vi "set_ready.vi"(8 "error in (no error)":errorcluster, 10 "ready?":bool, 11 "ErrorController in":refnum<class "ErrorController.lvclass">) -> (0 "error out":errorcluster, 3 "ErrorController out":refnum<class "ErrorController.lvclass">)   [LabVIEW 2010, in "ErrorController.lvclass"]
uses:
  ErrorController.lvclass
  ErrorController.lvclass/ErrorController.ctl
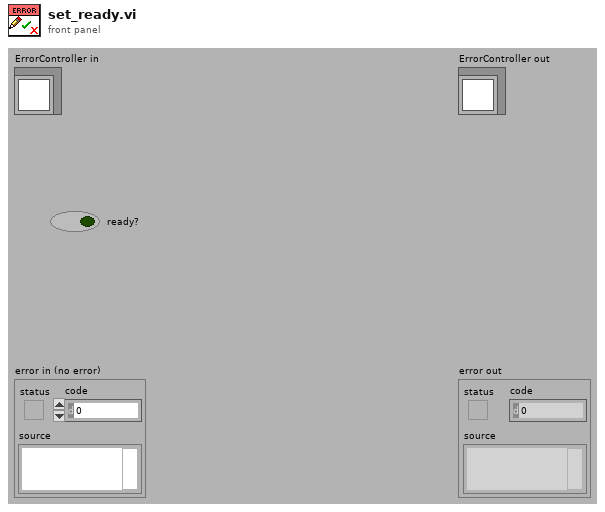
[diagram p1: front panel]
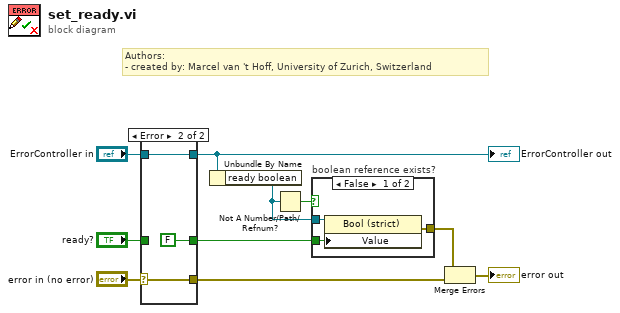
[diagram p0: block diagram]
diagram:
  # "Authors: \n- created by: Marcel van 't Hoff, University of Zurich, Switzerland"
  n1 = case shown="Error" "error in (no error)" {
    selector: "error in (no error)" -> [w12 w16]
    tunnel: [w12 w16] -> w1
    tunnel: [w13 w15] -> w7
    tunnel: "ErrorController in" -> [w13 w15]
    tunnel: [w11 FALSE ("ready?")] -> w4
    tunnel: "ready?" -> [w11 _]
    frame No Error {
    }
    frame Error {
    }
  }
  "ErrorController out" <- w7
  n2 = Unbundle By Name(w7) -> ("ready boolean"=w5:refnum<vi>)
  n3 = Not A Number/Path/Refnum?(number/path/refnum=w5) -> (NaN/Path/Refnum?=w6:bool)
  n4 = case "boolean reference exists?" shown="False" w6 {
    tunnel: w4 -> [w19 _]
    tunnel: [w18 _] -> w3
    tunnel: w5 -> [w17 _]
    frame False {
      n5 = property class="Bool (strict)"(reference=w17, "Value"=w19) -> (error out=w18:errorcluster)  [unwired: 1 in, 1 out]
    }
    frame True {
    }
  }
  n6 = Merge Errors(w3, w1) -> (→"error out":errorcluster)
